vi "Close Caller FP if In LabVIEW folder.vi"(7 "reference":refnum<vi>, 8 "error in (no error)":errorcluster) -> (0 "error out":errorcluster)   [LabVIEW 2017, in "_Try Beta Version of CSMF.lvlib"]
uses:
  _Try Beta Version of CSMF.lvlib
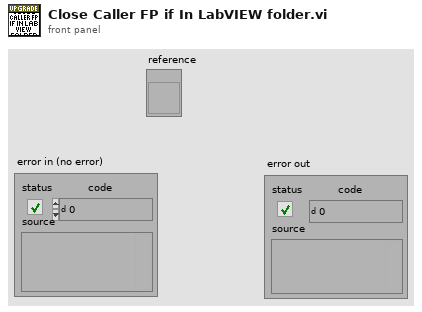
[diagram p1: front panel]
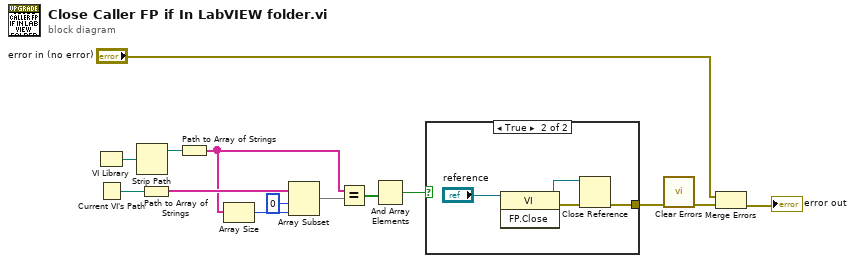
[diagram p0: block diagram]
diagram:
  n1 = VI Library() -> (path=w13:path)
  n2 = Current VI's Path() -> (path=w11:path)
  n3 = Strip Path(path=w13) -> (stripped path=w12:path)  [unwired: 1 out]
  n4 = Path to Array of Strings(0:w11) -> (2:w10:string[])  [unwired: 1 out]
  n5 = Path to Array of Strings(0:w12) -> (2:w6:string[])  [unwired: 1 out]
  n6 = Array Size(array=w6) -> (size(s)=w9:i32)
  n7 = Array Subset(array=w10, index=0, length=w9) -> (w7:string[])
  n8 = Equal?(x=w6, y=w7) -> (x = y?=w5:bool[])
  n9 = And Array Elements(Boolean array=w5) -> (logical AND=w4:bool)
  n10 = case shown="True" w4 {
    tunnel: [_ w17] -> w14
    frame False {
    }
    frame True {
      n11 = invoke class="VI" method="FP.Close"(reference="reference") -> (reference out=w16:refnum<vi>, error out=w18:errorcluster)  [unwired: 2 in, 1 out]
      n12 = Close Reference(reference=w16, error in (no error)=w18) -> (error out=w17:errorcluster)
    }
  }
  n13 = call <vilib>:"Clear Errors.vi"("error in (no error)"=w14) -> ("error out"=w1:errorcluster)  [unwired: 5 in, 1 out]
  n14 = Merge Errors("error in (no error)", w1) -> (→"error out":errorcluster)
